vi "TwoButtons Dialog.vi"(4 "ButtonTextCancel":string="Abbrechen", 6 "ButtonTextOK":string="OK", 8 "error in (no error)":errorcluster, 11 "Message":string) -> (0 "error out":errorcluster, 3 "OK?":bool)   [LabVIEW 2020]
uses:
  <vilib>/MGI/Panel Manager/Panel/Panel.lvlib
  <vilib>/MGI/Panel Manager/Panel/Panel/Panel.lvclass
  <vilib>/MGI/Panel Manager/Panel/Panel/Window/Dialog/Dialog.vi
  <vilib>/MGI/Panel Manager/Panel/Panel/Window/Dialog/Dialog.lvclass
  C:/Program Files (x86)/National Instruments/LabVIEW 2023/vi.lib/MGI/Panel Manager/Panel/Panel/Panel.lvclass
panel:
  in  "ButtonCancel?":bool
  in  "ButtonOK?":bool
  out "MessageText":string
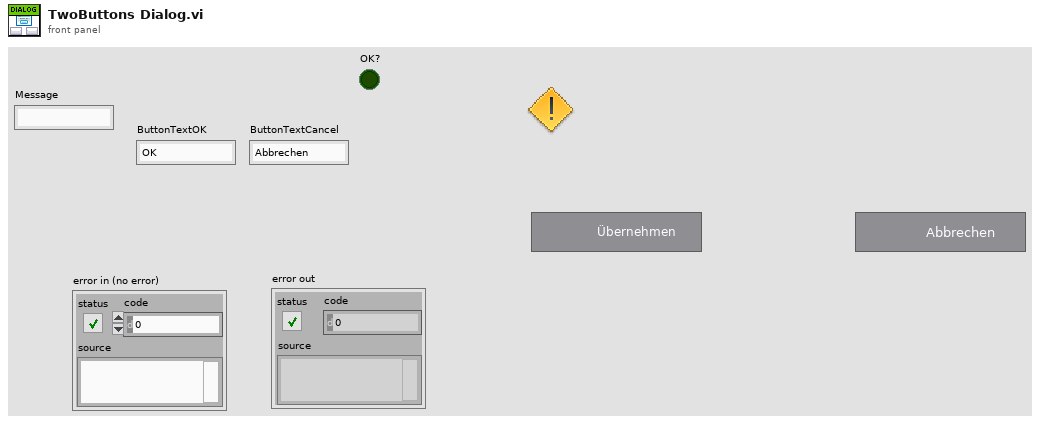
[diagram p1: front panel]
types:
  T1 = typedef "eventvkey.ctl" = enum16{"ASCII", "Enter", "Return", "Shift", "Ctrl", "Alt", "Cmd", "Opt", "Caps", "NumLock", "Clear", "Break", "Up", "Down", "Left", "Right", "Insert", "Delete", "Home", "End", "PageUp", "PageDown", "Escape", "Help", "Pause", "ScrollLock", "F1", "F2", "F3", "F4", "F5", "F6", "F7", "F8", "F9", "F10", "F11", "F12", "F13", "F14", "F15", "F16", "F17", "F18", "F19", "F20", "F21", "F22", "F23", "F24", "Play", "VolumeUp", "VolumeDown", "Mute", "Two Byte Char"}
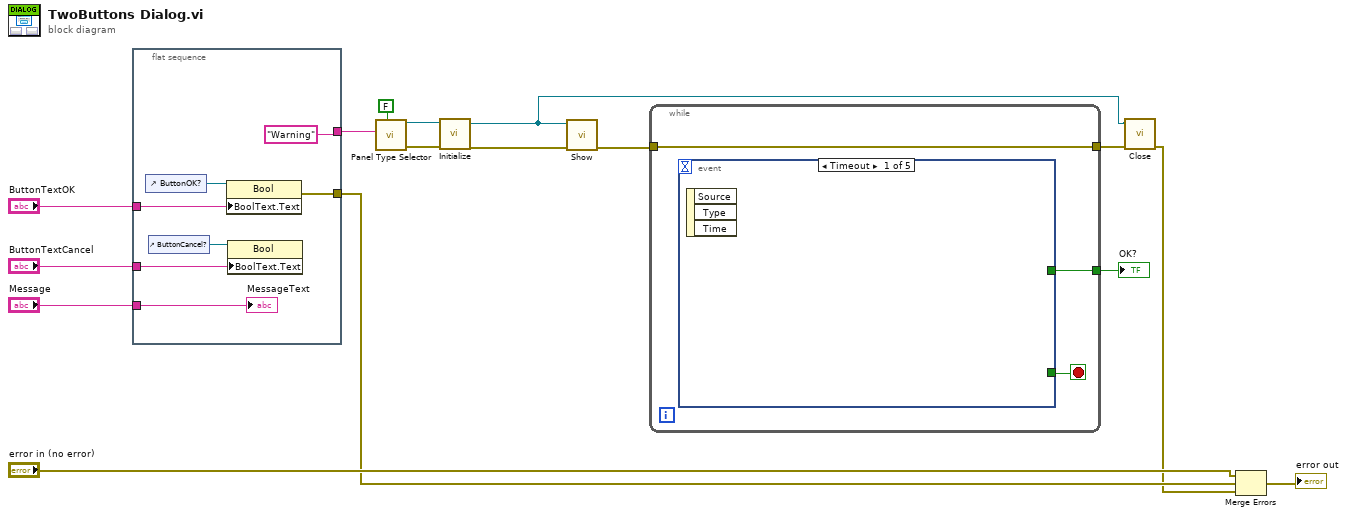
[diagram p0: block diagram]
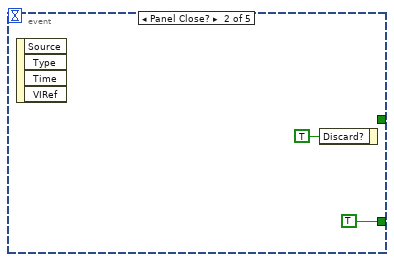
[diagram p2: hidden frame]
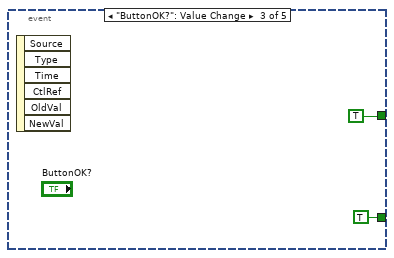
[diagram p3: hidden frame]
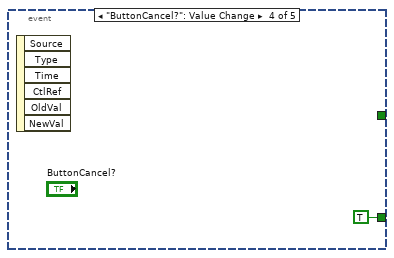
[diagram p4: hidden frame]
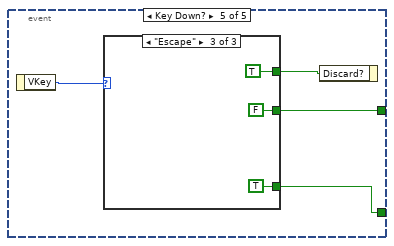
[diagram p5: hidden frame]
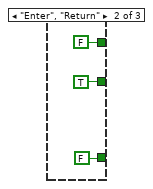
[diagram p7: hidden frame]
diagram:
  n1 = flat-sequence {
    tunnel: "ButtonTextOK" -> [w23]
    tunnel: "Message" -> [w22]
    tunnel: [w21] -> w12
    tunnel: ["Warning"] -> w11
    tunnel: "ButtonTextCancel" -> [w20]
    frame #0 {
      n2 = control-ref of="ButtonOK?"() -> (w18:refnum<vi>)
      n3 = control-ref of="ButtonCancel?"() -> (w19:refnum<vi>)
      n4 = property class="Bool"(reference=w18, "BoolText.Text"=w23) -> (error out=w21:errorcluster)  [unwired: 1 in, 1 out]
      n5 = property class="Bool"(reference=w19, "BoolText.Text"=w20) -> ()  [unwired: 1 in, 2 out]
      "MessageText" <- w22
    }
  }
  n6 = call-poly <vilib>:"Panel Type Selector.vi"("Autoshow? (T)"=FALSE, "Default Title"=w11) -> ("Error Out"=w9:errorcluster, "Dialog out"=w10:refnum<class "Dialog.lvclass">)  [unwired: 8 in]
  n7 = call <vilib>:"Initialize.vi"("error in (no error)"=w9, "Panel In"=w10) -> ("error out"=w5:errorcluster, "Panel Out"=w6:refnum<class "Dialog.lvclass">)  [unwired: 7 in, 1 out]
  n8 = call <vilib>:"Show.vi"("Error In"=w5, "Panel in"=w6) -> ("Error Out"=w4:errorcluster)  [unwired: 9 in]
  n9 = while {
    tunnel: [w26] -> w7
    tunnel: w4 -> [w26]
    tunnel: [w24] -> w2
    stop <- w25 stop-if-true
    n10 = event shown="[0] Timeout" {
      selector: _ -> [_ _ _ _ _]
      dyn-events: _ -> [_ _ _ _ _]
      timeout: _ -> [_ _ _ _ _]
      tunnel: [_ TRUE ("Discard?") TRUE ("Discard?") TRUE ("Discard?") w32] -> w25
      tunnel: [_ _ TRUE _ w33] -> w24
      event Timeout {
        n11 = event-data() -> ()  [unwired: 1 in, 3 out]
      }
      event Panel Close? {
        n12 = event-data() -> ()  [unwired: 1 in, 4 out]
        n13 = event-data("Discard?"=TRUE) -> ()  [unwired: 1 in, 1 out]
      }
      event "ButtonOK?": Value Change {
        n14 = event-data() -> ()  [unwired: 1 in, 6 out]
      }
      event "ButtonCancel?": Value Change {
        n15 = event-data() -> ()  [unwired: 1 in, 6 out]
      }
      event Key Down? {
        n16 = event-data() -> ("VKey"=w35:T1)  [unwired: 1 in]
        n17 = case shown="\"Escape\"" w35 {
          tunnel: [_ FALSE ("Discard?") TRUE ("Discard?")] -> w34
          tunnel: [_ TRUE FALSE] -> w33
          tunnel: [_ FALSE TRUE] -> w32
          frame "ASCII", Default {
          }
          frame "Enter", "Return" {
          }
          frame "Escape" {
          }
        }
        n18 = event-data("Discard?"=w34) -> ()  [unwired: 1 in, 1 out]
      }
    }
  }
  "OK?" <- w2
  n19 = call-dynamic "Close.vi"("error in (no error)"=w7, "Dialog in"=w6) -> ("error out"=w8:errorcluster)  [unwired: 9 in]
  n20 = Merge Errors("error in (no error)", w12, w8) -> (→"error out":errorcluster)
